vi "TimerDummy.vi"() -> ()   [LabVIEW 2025]
uses:
  <userlib>/_OpenG.lib/comparison/comparison.llb/Boolean Changed__ogtk.vi
  <vilib>/NI/Timer/Timer Session.lvclass
  <userlib>/_OpenG.lib/comparison/comparison.llb/openg_comparison__ogtk.lvlib
panel:
  in  "Boolean":bool
  out "Elapsed Time":dbl
  in  "stop":bool
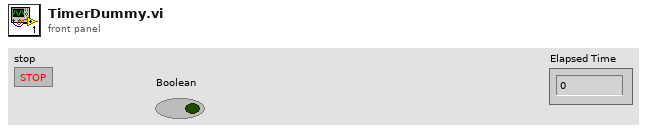
[diagram p1: front panel]
types:
  T1 = typedef "Timer Session.lvclass/Session Handle.ctl" = refnum<data-value>
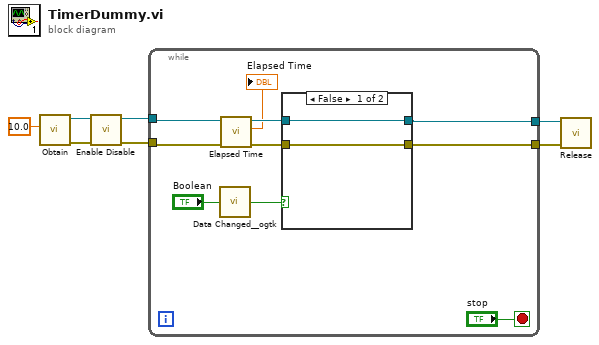
[diagram p0: block diagram]
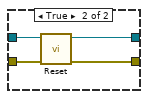
[diagram p2: hidden frame]
diagram:
  n1 = call <vilib>:"Obtain.vi"("Time Goal (s)"=10.0) -> ("Error Out"=w7:errorcluster, "Timer Handle"=w6:T1)  [unwired: 9 in]
  n2 = call <vilib>:"Enable Disable.vi"("Error In"=w7, "Timer Handle"=w6) -> ("Error Out"=w4:errorcluster, "Timer Handle"=w5:T1)  [unwired: 8 in]
  n3 = while {
    tunnel: w5 -> [w16]
    tunnel: w4 -> [w15]
    tunnel: [w11] -> w1
    tunnel: [w10] -> w2
    stop <- "stop" stop-if-true
    n4 = call-poly <userlib>:"Data Changed__ogtk.vi"("Boolean"="Boolean") -> ("Changed"=w8:bool)
    n5 = call <vilib>:"Elapsed Time.vi"("Error In"=w15, "Timer Handle"=w16) -> ("Error Out"=w14:errorcluster, "Elapsed Time"=→"Elapsed Time":dbl, "Timer Handle"=w13:T1)  [unwired: 6 in, 1 out]
    n6 = case shown="False" w8 {
      tunnel: w14 -> [w18 w23]
      tunnel: w13 -> [w19 w22]
      tunnel: [w18 w21] -> w10
      tunnel: [w19 w20] -> w11
      frame False {
      }
      frame True {
        n7 = call <vilib>:"Reset.vi"("Error In"=w23, "Timer Handle"=w22) -> ("Error Out"=w21:errorcluster, "Timer Handle"=w20:T1)  [unwired: 8 in]
      }
    }
  }
  n8 = call <vilib>:"Release.vi"("Error In"=w2, "Timer Handle"=w1) -> ()  [unwired: 8 in, 2 out]
